vi "GetStatusRegisterFormat.vi"(8 "Error In":errorcluster, 11 "Keithley 6482 In":refnum<visa-resource-name>) -> (0 "Error Out":errorcluster, 2 "Status Register Format":T1, 3 "Keithley 6482 Out":refnum<visa-resource-name>)   [LabVIEW 8.6, in "Keithley-6482-Visa.lvlib"]
uses:
  Keithley-6482-Visa.lvlib
  Controls/StatusRegisterFormat.ctl
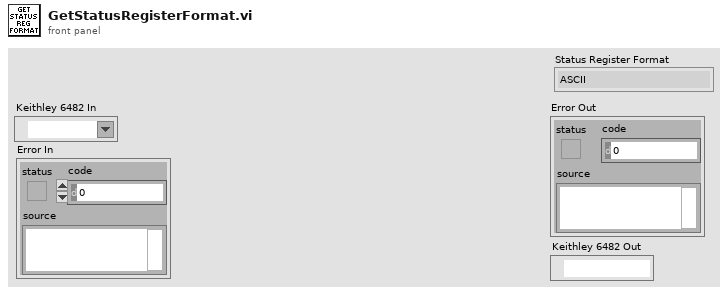
[diagram p1: front panel]
types:
  T1 = typedef "Keithley-6482-Visa.lvlib/StatusRegisterFormat.ctl" = enum16{"ASCII", "Hexadecimal", "Octal", "Binary"}
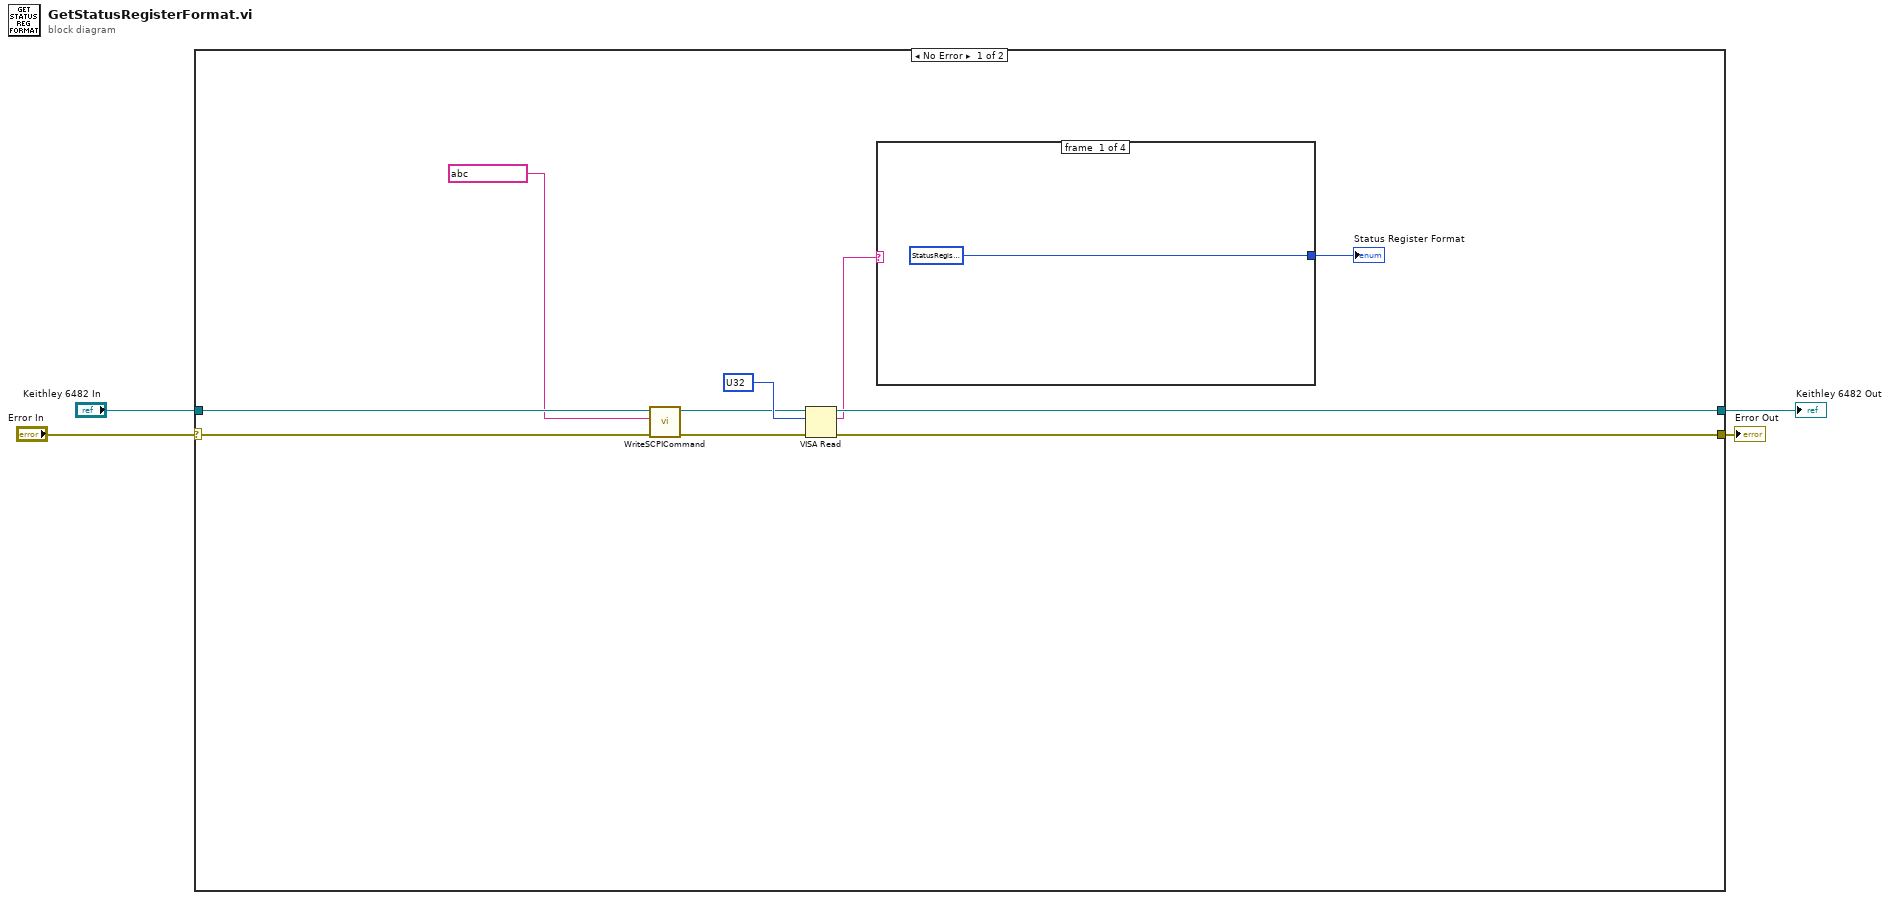
[diagram p0: block diagram]
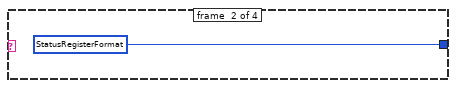
[diagram p2: hidden frame]
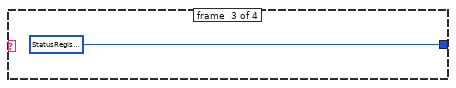
[diagram p3: hidden frame]
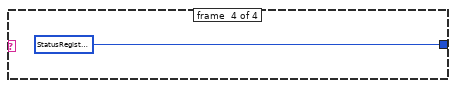
[diagram p4: hidden frame]
diagram:
  n1 = case shown="No Error" "Error In" {
    selector: "Error In" -> [w7 w19]
    tunnel: "Keithley 6482 In" -> [w6 w20]
    tunnel: [w14 w19] -> w2
    tunnel: [w13 w20] -> w1
    frame #0 {
      n2 = call "WriteSCPICommand.vi"("Error In"=w7, "SCPI Command"=string ?, "Keithley 6482 In"=w6) -> ("Error Out"=w8:errorcluster, "Keithley 6482 Out"=w9:refnum<visa-resource-name>)  [unwired: 7 in]
      n3 = VISA Read(VISA resource name=w9, byte count=u32 ?, error in (no error)=w8) -> (VISA resource name out=w13:refnum<visa-resource-name>, read buffer=w11:string, error out=w14:errorcluster)  [unwired: 1 out]
      n4 = case shown="\"BIN\"" w11 {
        tunnel: [T1 ? ("Status Register Format") T1 ? ("Status Register Format") T1 ? ("Status Register Format") T1 ? ("Status Register Format")] -> w10
        frame #0 {
        }
        frame #1 {
        }
        frame #2 {
        }
        frame #3 {
        }
      }
      "Status Register Format" <- w10
    }
    frame #1 {
    }
  }
  "Error Out" <- w2
  "Keithley 6482 Out" <- w1
